vi "ABCD.vi"(9 "z":dbl format="%#_13g", 10 "y":dbl, 11 "x":dbl) -> (0 "D":dbl, 1 "C":dbl, 2 "B":dbl, 3 "A":dbl)   [LabVIEW 2019]
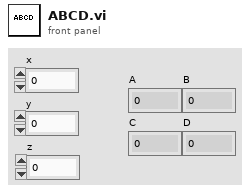
[diagram p1: front panel]
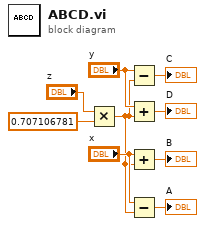
[diagram p0: block diagram]
diagram:
  n1 = Multiply(x="z", y=0.707106781) -> (x*y=w2:dbl)
  n2 = Subtract(x="y", y=w2) -> (x-y=→"C":dbl)
  n3 = Add(x="y", y=w2) -> (x+y=→"D":dbl)
  n4 = Add(x="x", y=w2) -> (x+y=→"B":dbl)
  n5 = Subtract(x="x", y=w2) -> (x-y=→"A":dbl)
